vi "BRig_dataExp_Audio_freq_1B.vi"() -> (2 "output_Audio_freq__1B":i32)   [LabVIEW 2014]
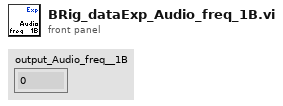
[diagram p1: front panel]
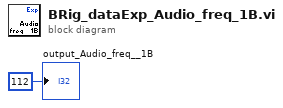
[diagram p0: block diagram]
diagram:
  "output_Audio_freq__1B" <- 112 ("output_iBlock")
